vi "NI VeriStand - Remove Custom Device Item.vi"(8 "error in (no error)":errorcluster, 10 "Force Delete (F)":bool, 11 "Item Ref in":T1 format="%.0x") -> (0 "error out":errorcluster, 2 "Deleted?":bool)   [LabVIEW 2026, in "Custom Devices Storage.lvlib"]
uses:
  Custom Devices Storage.lvlib
  <vilib>/NI VeriStand/Custom Device API/Custom Device Item Ref.ctl
  <vilib>/NI VeriStand/Custom Device API/Custom Device API.lvlib
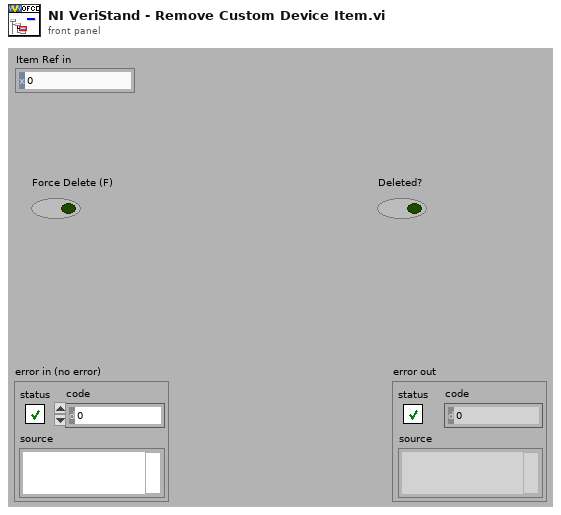
[diagram p1: front panel]
types:
  T1 = typedef "Custom Device API.lvlib/Custom Device Item Ref.ctl" = u64
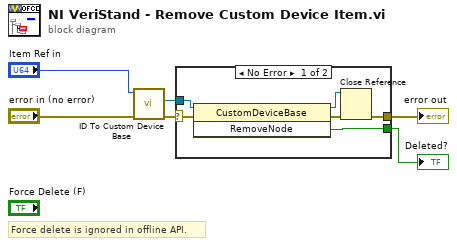
[diagram p0: block diagram]
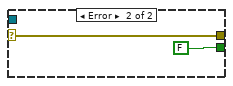
[diagram p2: hidden frame]
diagram:
  # "Force delete is ignored in offline API."
  n1 = call "ID To Custom Device Base.vi"("error in (no error)"="error in (no error)", "ID in"="Item Ref in") -> ("error out"=w1:errorcluster, "BaseNode"=w4:refnum<k39>)  [unwired: 7 in, 1 out]
  n2 = case shown="No Error" w1 {
    selector: w1 -> [w7 w14]
    tunnel: w4 -> [w12 _]
    tunnel: [w11 FALSE ("RemoveNode")] -> w3
    tunnel: [w8 w14] -> w2
    frame No Error {
      n3 = invoke class="CustomDeviceBase" method="RemoveNode"(reference=w12, error in=w7) -> (reference out=w9:refnum<k39>, error out=w10:errorcluster, "RemoveNode"=w11:bool)  [unwired: 1 in]
      n4 = Close Reference(reference=w9, error in (no error)=w10) -> (error out=w8:errorcluster)
    }
    frame Error {
    }
  }
  "error out" <- w2
  "Deleted?" <- w3
